vi "create complex single tone signal.vi"(6 "sampling info":cluster{"Fs":dbl, "#s":dbl}={"Fs"=1000.0, "#s"=1000.0}, 8 "Noise level":dbl, 9 "phase (deg)":dbl, 10 "amplitude":dbl=1.0, 11 "frequency (Hz)":dbl=10.0) -> (3 "complex waveform":waveform(cdb))   [LabVIEW 2023]
doc: "Create complex single-tone signal."
uses:
  <vilib>/Analysis/NI_AALBase.lvlib
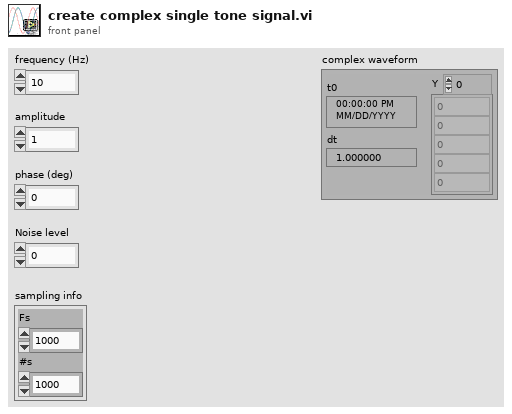
[diagram p1: front panel]
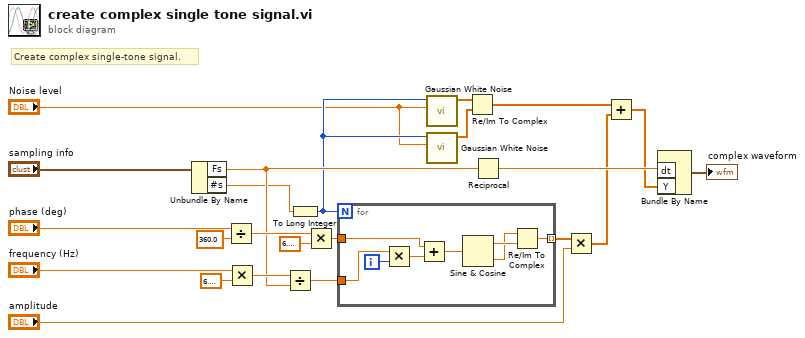
[diagram p0: block diagram]
diagram:
  # "Create complex single-tone signal."
  n1 = Unbundle By Name("sampling info") -> ("Fs"=w9:dbl, "#s"=w8:dbl)
  n2 = Divide(x="phase (deg)", y=360.0) -> (x/y=w21:dbl)
  n3 = Multiply(x="frequency (Hz)", y=6.283185307179586) -> (x*y=w17:dbl)
  n4 = Divide(x=w17, y=w9) -> (x/y=w16:dbl)
  n5 = To Long Integer(number=w8) -> (32bit integer=w6:i32)
  n6 = Multiply(x=w21, y=6.283185307179586) -> (x*y=w15:dbl)
  n7 = for {
    N: w6 -> [_]
    tunnel: w16 -> [w30]
    tunnel: w15 -> [w28]
    tunnel: [w27] -> w13 mode=indexing
    i -> [w31]
    n8 = Multiply(x=w30, y=w31) -> (x*y=w29:dbl)
    n9 = Add(x=w28, y=w29) -> (x+y=w26:dbl)
    n10 = Sine & Cosine(0:w26) -> (1:w25:dbl, 2:w24:dbl)
    n11 = Re/Im To Complex(1:w25, 2:w24) -> (0:w27:cdb)
  }
  n12 = call <vilib>:"Gaussian White Noise.vi"("standard deviation"="Noise level", "samples"=w6) -> ("Gaussian noise pattern"=w4:dbl[])  [unwired: 2 in, 7 out]
  n13 = call <vilib>:"Gaussian White Noise.vi"("standard deviation"="Noise level", "samples"=w6) -> ("Gaussian noise pattern"=w3:dbl[])  [unwired: 2 in, 7 out]
  n14 = Re/Im To Complex(1:w3, 2:w4) -> (0:w2:cdb[])
  n15 = Reciprocal(x=w9) -> (1/x=w11:dbl)
  n16 = Multiply(x=w13, y="amplitude") -> (x*y=w7:cdb[])
  n17 = Add(x=w2, y=w7) -> (x+y=w1:cdb[])
  n18 = Bundle By Name("dt"=w11, "Y"=w1) -> (→"complex waveform":waveform(cdb))  [unwired: 1 out]
